vi "niDAQmx Get Task Property.vi"   [LabVIEW 2021, in "Session Management niDAQmx.lvlib" / "Session Factory.lvclass"]
doc: "Property node to get information from NI-DAQmx tasks."
uses:
  Session Factory.lvclass
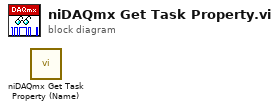
[diagram p0: block diagram]
diagram:
  n1 = call "niDAQmx Get Task Property (Name).vi"() -> ()  [unwired: 13 in, 3 out]
